vi "Read RoleRef.vi"(8 "error in (no error)":errorcluster, 11 "Play in":refnum<class "Play.lvclass">) -> (0 "error out":errorcluster, 2 "RoleRef":refnum<class "Role.lvclass">[](array[class]), 3 "Play out":refnum<class "Play.lvclass">)   [LabVIEW 2018, in "Play.lvclass"]
uses:
  Play.lvclass
  Role_class/Role.lvclass
  Play.lvclass/Play.ctl
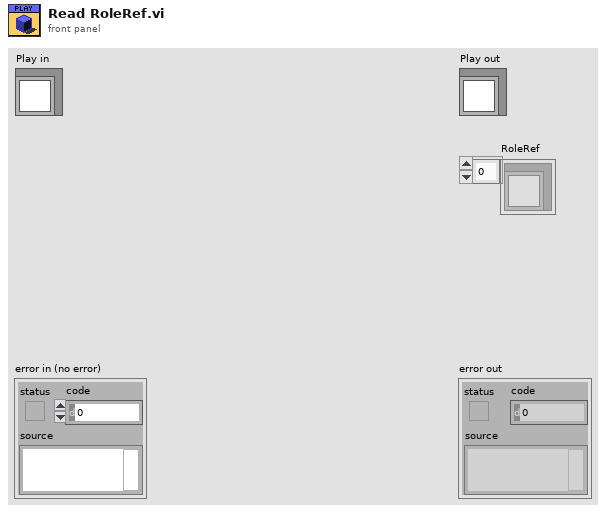
[diagram p1: front panel]
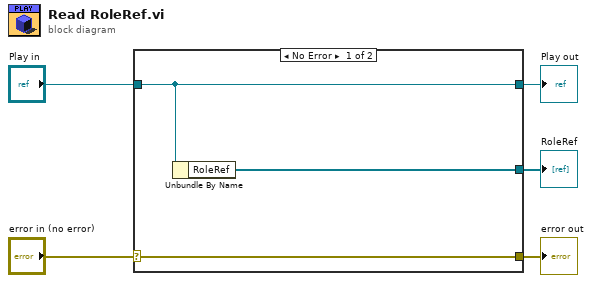
[diagram p0: block diagram]
diagram:
  n1 = case shown="No Error" "error in (no error)" {
    selector: "error in (no error)" -> [w8 w9]
    tunnel: [w8 w9] -> w4
    tunnel: [w7 w10] -> w2
    tunnel: "Play in" -> [w7 w10]
    tunnel: [w6 _] -> w1
    frame No Error {
      n2 = Unbundle By Name(w7) -> ("RoleRef"=w6:refnum<class "Role.lvclass">[])
    }
    frame Error {
    }
  }
  "error out" <- w4
  "Play out" <- w2
  "RoleRef" <- w1
